vi "AlliGator Create Gate Image if needed.vi"(6 "Image Characteristics":T2 {"Calibration"."Y Step" format="%.2f"; "Calibration"."X Step" format="%.2f"; "Image Type" items=["Grayscale (U8)", "Grayscale (I16)", "Grayscale (SGL)", "Complex (CSG)", "RGB (U32)", "HSL (U32)", "RGB (U64)", "Grayscale (U16)"]}, 7 "Prefix String":string, 8 "error in (no error)":errorcluster, 9 "Gate ID":string, 10 "Image Reused?":bool, 11 "Gate Image":T1) -> (0 "error out":errorcluster, 1 "Number of Created Images":i32, 2 "Image available?":bool, 3 "Gate Image":T1)   [LabVIEW 2021, in "AlliGator Files.lvlib"]
doc: "Creates an image structure if needed."
uses:
  AlliGator Files.lvlib
  Image/Image Characteristics.ctl
  <vilib>/vision/Image Controls.llb/IMAQ Image.ctl
  Error/Error.lvlib
  Image/Image.lvlib
panel:
  # "see the AlliGator License on the block diagram (Ctrl+E or Window:Show Block Diagram)"
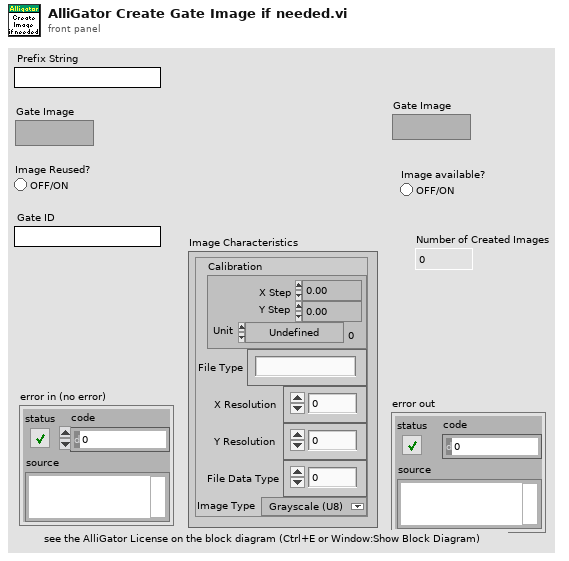
[diagram p1: front panel]
types:
  T1 = typedef "IMAQ Image.ctl" = refnum<image>
  T2 = typedef "Image.lvlib/Image Characteristics.ctl" = cluster{"Calibration":T3, "File Type":string, "X Resolution":i32, "Y Resolution":i32, "File Data Type":i32, "Image Type":T5}
  T3 = typedef "Simple Grid Descriptor" = cluster{"X Step":sgl, "Y Step":sgl, "Unit":T4}
  T4 = typedef "Image Unit" = enum32{"Undefined", "Angström", "Micrometer", "Millimeter", "Centimeter", "Meter", "Kilometer", "Microinch", "Inch", "Feet", "Nautical miles", "Standard miles", "Steps"}
  T5 = typedef "Image Type" = u32
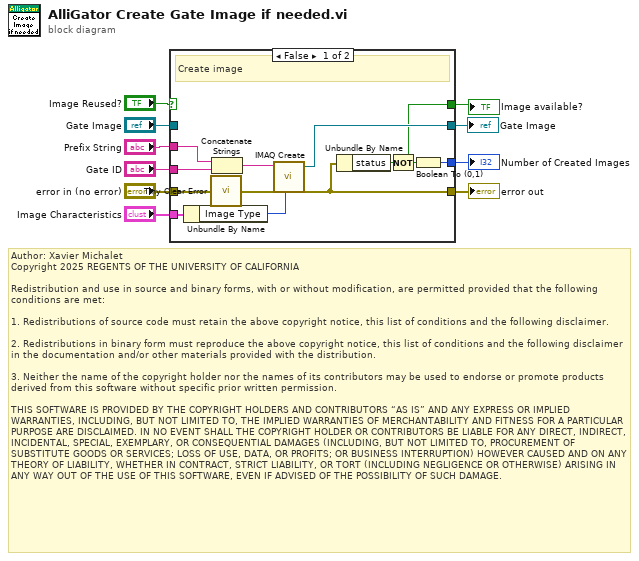
[diagram p0: block diagram]
diagram:
  # "Author: Xavier Michalet\nCopyright 2025 REGENTS OF THE UNIVERSITY OF CALIFORNIA\n\nRedistribution and use in source and binary forms, with or without modification, are permitted provided that the following conditions are met:\n\n1. Redistributions of source code must retain the above copyright notice, this list of conditions and the following disclaimer.\n\n2. Redistributions in binary form must reproduce the above copyright notice, this list of conditions and the following disclaimer in the documentation and/or other materials provided with the distribution.\n\n3. Neither the name of the copyright holder nor the names of its contributors may be used to endorse or promote products derived from this software without specific prior written permission.\n\nTHIS SOFTWARE IS PROVIDED BY THE COPYRIGHT HOLDERS AND CONTRIBUTORS “AS IS” AND ANY EXPRESS OR IMPLIED WARRANTIES, INCLUDING, BUT NOT LIMITED TO, THE IMPLIED WARRANTIES OF MERCHANTABILITY AND FITNESS FOR A PARTICULAR PURPOSE ARE DISCLAIMED. IN NO EVENT SHALL THE COPYRIGHT HOLDER OR CONTRIBUTORS BE LIABLE FOR ANY DIRECT, INDIRECT, INCIDENTAL, SPECIAL, EXEMPLARY, OR CONSEQUENTIAL DAMAGES (INCLUDING, BUT NOT LIMITED TO, PROCUREMENT OF SUBSTITUTE GOODS OR SERVICES; LOSS OF USE, DATA, OR PROFITS; OR BUSINESS INTERRUPTION) HOWEVER CAUSED AND ON ANY THEORY OF LIABILITY, WHETHER IN CONTRACT, STRICT LIABILITY, OR TORT (INCLUDING NEGLIGENCE OR OTHERWISE) ARISING IN ANY WAY OUT OF THE USE OF THIS SOFTWARE, EVEN IF ADVISED OF THE POSSIBILITY OF SUCH DAMAGE."
  n1 = case shown="False" "Image Reused?" {
    selector: "Image Reused?" -> [_ w23]
    tunnel: [w19 w24] -> w8
    tunnel: [w22 w25] -> w7
    tunnel: "error in (no error)" -> [w21 w24]
    tunnel: "Gate ID" -> [w20 _]
    tunnel: "Gate Image" -> [_ w25]
    tunnel: [w12 _] -> w2
    tunnel: "Prefix String" -> [w15 _]
    tunnel: "Image Characteristics" -> [w14 _]
    tunnel: [w11 w23] -> w1
    frame False {
      # "Create image"
      n2 = Unbundle By Name(w14) -> ("Image Type"=w13:T5)
      n3 = call "Tiny Clear Error.vi"("Error In"=w21) -> ("no Error Out"=w17:errorcluster)  [unwired: 8 in]
      n4 = Concatenate Strings(w15, w20) -> (w16:string)
      n5 = call "IMAQ Create"("Image Name"=w16, "Image Type"=w13, "error in (no error)"=w17) -> ("New Image"=w22:T1, "error out"=w19:errorcluster)  [unwired: 2 in]
      n6 = Unbundle By Name(w19) -> ("status"=w18:bool)
      n7 = Not(x=w18) -> (.not. x?=w11:bool)
      n8 = Boolean To (0,1)(Boolean=w11) -> (0, 1=w12:i16)
    }
    frame True {
    }
  }
  "error out" <- w8
  "Gate Image" <- w7
  "Number of Created Images" <- w2
  "Image available?" <- w1
